vi "Configure Control.vi"   [LabVIEW 2020, in "PV Access.lvlib" / "PV Data.lvlib" / "NT Scalar (Numeric).lvclass"]
uses:
  NT Scalar (Numeric).lvclass
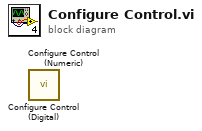
[diagram p0: block diagram]
diagram:
  n1 = call "Configure Control (Digital).vi"() -> ()  [unwired: 9 in, 3 out]
  n2 = call "Configure Control (Numeric).vi"() -> ()  [unwired: 9 in, 3 out]
